vi "Get Data Client Wrapper.vi"(8 "error in":errorcluster, 11 "gRPC ID in":T1) -> (0 "error out":errorcluster, 2 "Payload":u8[](array[numeric]), 3 "gRPC ID out":T1)   [LabVIEW 2025, in "Automotive Ethernet Bus Monitor UI.lvlib"]
doc: "Send a GetData Request to the server from the client side."
uses:
  Automotive Ethernet Bus Monitor UI.lvlib
  <vilib>/gRPC/LabVIEW gRPC Library/Shared/grpcId.ctl
  OOB gRPC Client/RPC Messages/hwval_GenericRequest.ctl
  OOB gRPC Client/OOB gRPC Client.lvlib
  <vilib>/gRPC/LabVIEW gRPC Library/grpc-lvsupport-release.lvlib
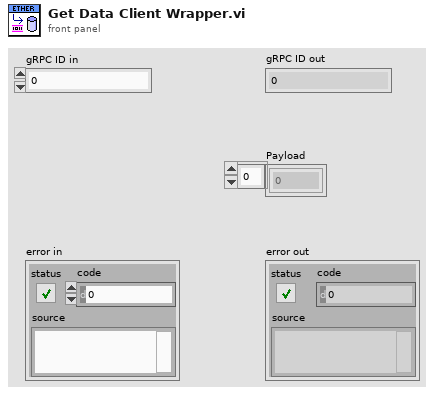
[diagram p1: front panel]
types:
  T1 = typedef "grpc-lvsupport-release.lvlib/grpcId.ctl" = u64
  T2 = typedef "OOB gRPC Client.lvlib/hwval_GenericRequest.ctl" = cluster{"Command":string, "Payload":u8[]}
  T3 = typedef "OOB gRPC Client.lvlib/hwval_GenericResponse.ctl" = cluster{"Payload":u8[]}
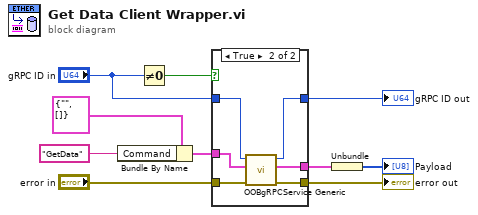
[diagram p0: block diagram]
diagram:
  n1 = Bundle By Name(cluster=T2 {"Command"="", "Payload"=[]} ("Request Data"), "Command"="GetData") -> (w4:T2)
  n2 = Not Equal To 0?(x="gRPC ID in") -> (x != 0?=w2:bool)
  n3 = case shown="True" w2 {
    tunnel: "gRPC ID in" -> [w11 w18]
    tunnel: [_ w17] -> w7
    tunnel: w4 -> [_ w16]
    tunnel: [w12 w15] -> w9
    tunnel: "error in" -> [w12 w14]
    tunnel: [w11 w13] -> w1
    frame False {
    }
    frame True {
      n4 = call "OOBgRPCService Generic.vi"("error in"=w14, "Request Data"=w16, "gRPC ID"=w18) -> ("error out"=w15:errorcluster, "Response Data"=w17:T3, "gRPC ID out"=w13:T1)  [unwired: 6 in]
    }
  }
  "error out" <- w9
  "gRPC ID out" <- w1
  n5 = Unbundle(w7) -> ("Payload"=→"Payload":u8[])
